vi "Password Authentication.vi"(8 "error in (no error)":errorcluster, 10 "Key":i16, 11 "Top in":refnum<class "Top.lvclass">) -> (0 "error out":errorcluster, 3 "Top out":refnum<class "Top.lvclass">)   [LabVIEW 2021, in "Top.lvlib" / "Top.lvclass"]
uses:
  Top.lvclass
  Top.lvclass/Top.ctl
  <vilib>/MGI/Panel Manager/Panel Actor/Panel Actor Messages/Show Panel Msg/Show Panel Msg.lvclass
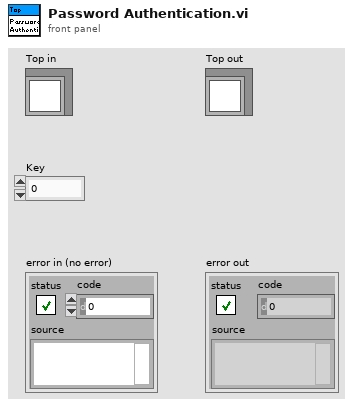
[diagram p1: front panel]
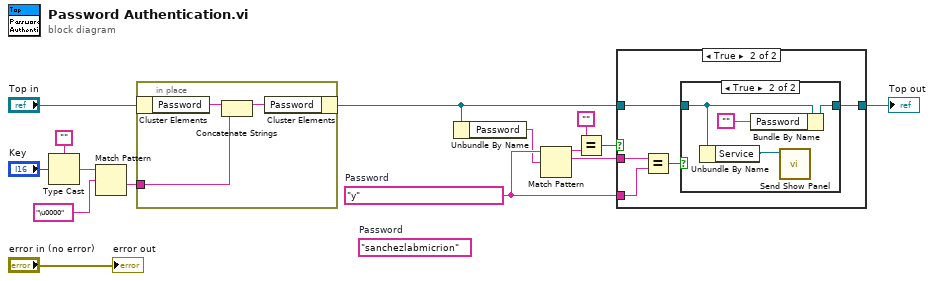
[diagram p0: block diagram]
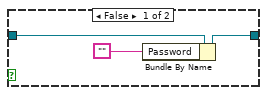
[diagram p2: hidden frame]
diagram:
  (unwired) "sanchezlabmicrion"  # Password
  w4 = "y"  # Password
  n1 = Type Cast(type="", x="Key") -> (*(type *) &x=w6:string)
  n2 = Match Pattern(string=w6, regular expression="\u0000") -> (after substring=w5:string)  [unwired: 1 in, 3 out]
  n3 = in-place {
    in-place-border: w5 -> [w16]
    n4 = in-place-cluster #1("Top in") -> ("Password"=w18:string)
    n5 = Concatenate Strings(w18, w16) -> (w17:string)
    n6 = in-place-cluster #1("Password"=w17) -> (w11:refnum<class "Top.lvclass">)
  }
  n7 = Unbundle By Name(w11) -> ("Password"=w3:string)
  n8 = Match Pattern(string=w4, regular expression=w3) -> (before substring=w2:string, match substring=w9:string)  [unwired: 1 in, 2 out]
  n9 = Equal?(x="", y=w2) -> (x = y?=w8:bool)
  n10 = case shown="True" w8 {
    tunnel: w11 -> [w21 w26]
    tunnel: [w20 w25] -> w10
    tunnel: w9 -> [_ w22]
    tunnel: w4 -> [_ w23]
    frame False {
      n11 = Bundle By Name(cluster=w21, "Password"="") -> (w20:refnum<class "Top.lvclass">)
    }
    frame True {
      n12 = Equal?(x=w22, y=w23) -> (x = y?=w24:bool)
      n13 = case shown="True" w24 {
        tunnel: w26 -> [w27 w28]
        tunnel: [w27 w30] -> w25
        frame False {
        }
        frame True {
          n14 = Unbundle By Name(w28) -> ("Service"=w31:refnum<class "Message Enqueuer.lvclass">)
          n15 = Bundle By Name(cluster=w28, "Password"="") -> (w30:refnum<class "Top.lvclass">)
          n16 = call <vilib>:"Send Show Panel.vi"("Message Enqueuer in"=w31) -> ()  [unwired: 9 in, 2 out]
        }
      }
    }
  }
  "Top out" <- w10
  "error out" <- "error in (no error)"
